vi "RC_Generate_Full_Condition(s)_text.vi"(7 "Array index to show":i32=-1, 8 "error in (no error)":errorcluster, 9 "Array of conditions in":T1, 10 "Calibration parameters":T2 {"True frame time, s" format="%.10g"; "Disp. calibration info"."Speed, µl per ms" format="%.3g"; "True FPS" format="%.10g"; "Timing calibration sw/hw" format="%.10g"}, 11 "TreeControl ref in":refnum<vi>) -> (0 "error out":errorcluster, 3 "TreeControl ref out":refnum<vi>)   [LabVIEW 2018, in "Tracker.lvlib" / "Reward_Condition.lvclass"]
uses:
  Reward_Condition.lvclass
  Controls/CTL_Dispenser_calibration_info.ctl
  Tracker.lvlib
  Controls/CTL_Calibration_parameters.ctl
  Controls/RC_Array_of_Conditions.ctl
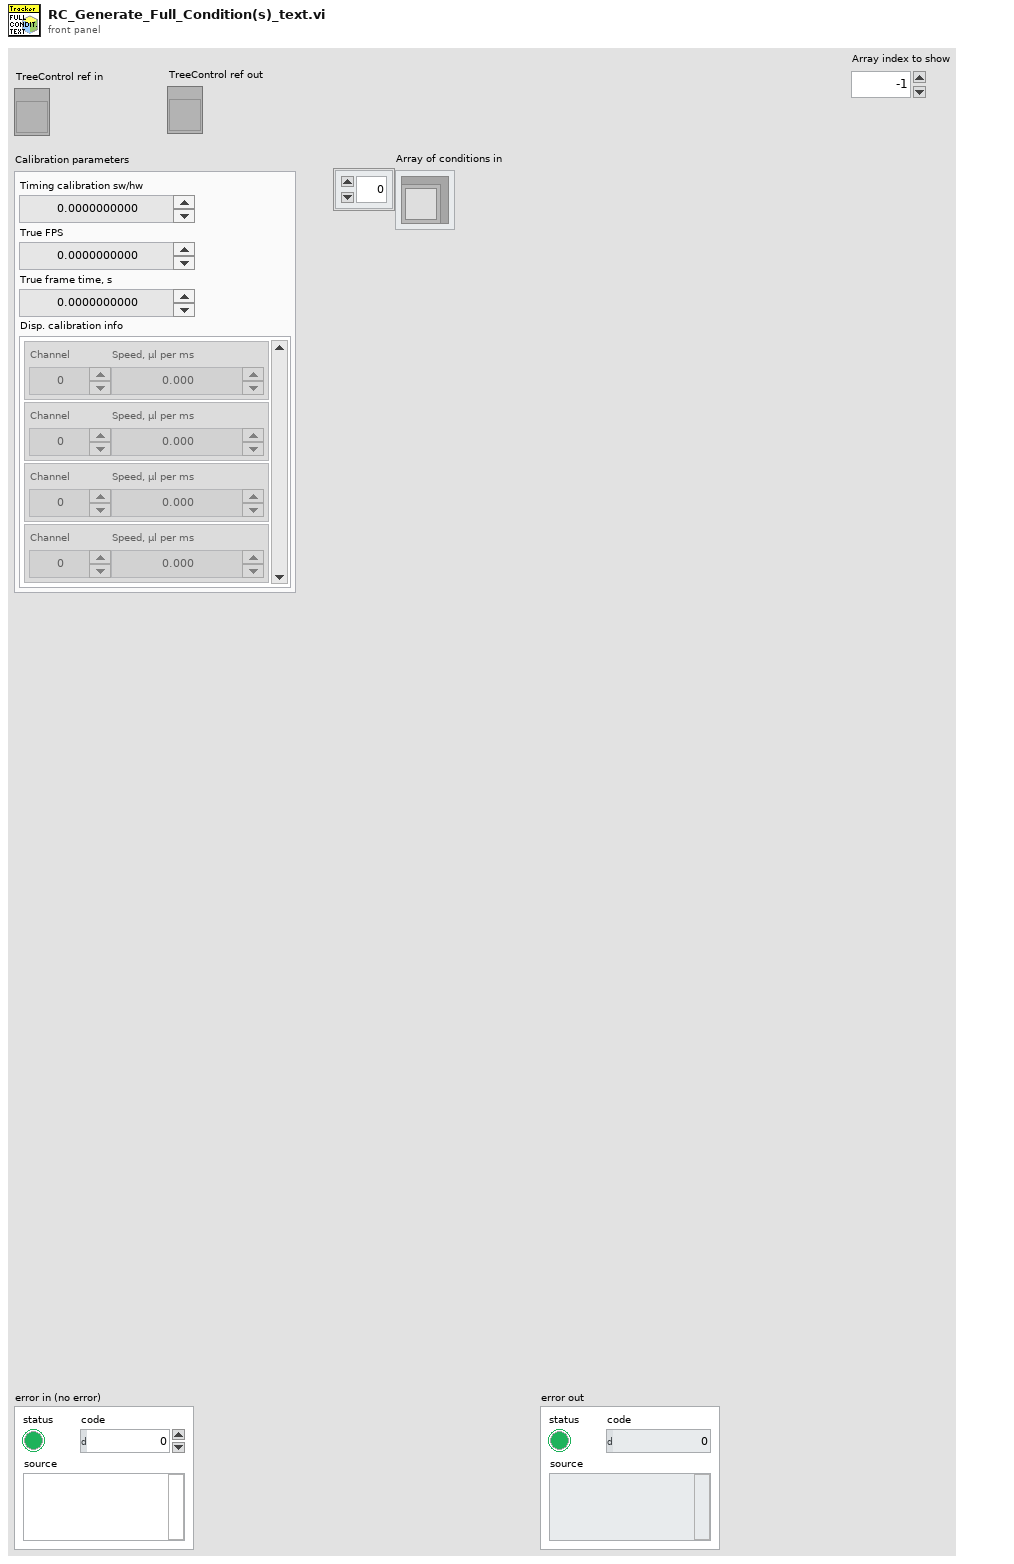
[diagram p1: front panel]
types:
  T1 = typedef "Tracker.lvlib/Reward_Condition.lvclass/RC_Array_of_Conditions.ctl" = refnum<class "Reward_Condition.lvclass">[]
  T2 = typedef "Tracker.lvlib/CTL_Calibration_parameters.ctl" = cluster{"Timing calibration sw/hw":dbl, "True FPS":dbl, "True frame time, s":dbl, "Disp. calibration info":T3}
  T3 = typedef "Tracker.lvlib/CTL_Dispenser_calibration_info.ctl" = cluster{"Channel":u8, "Speed, µl per ms":dbl}[]
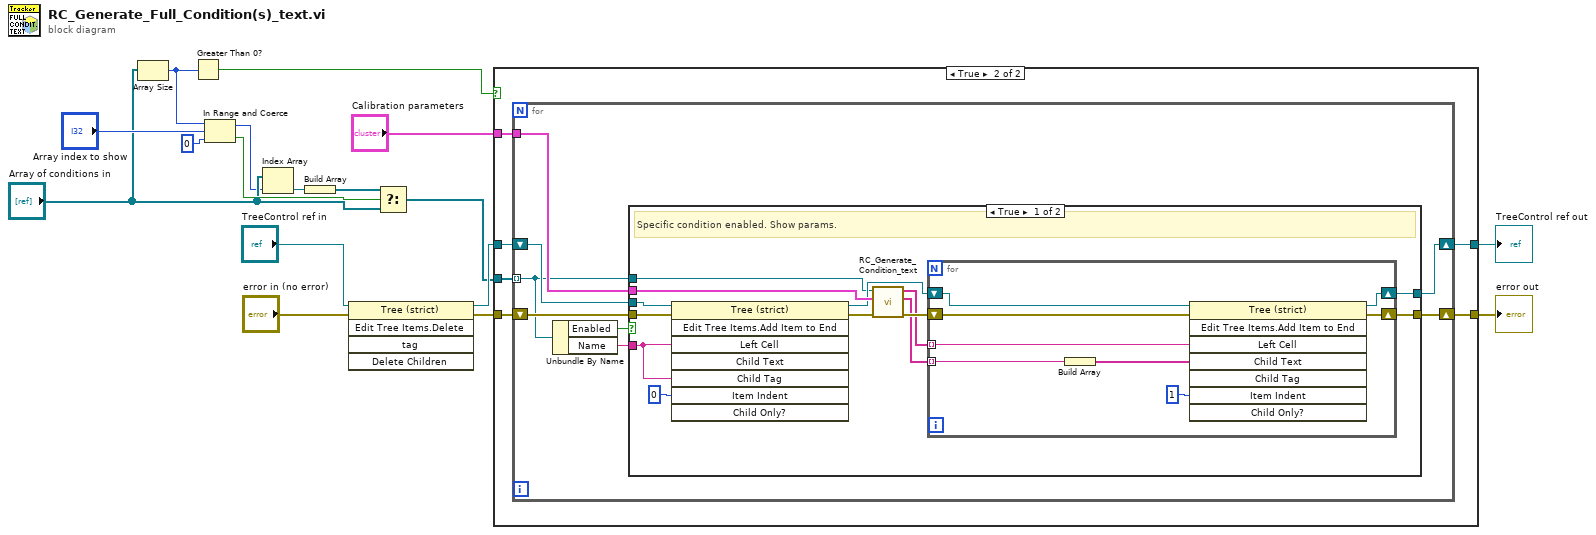
[diagram p0: block diagram]
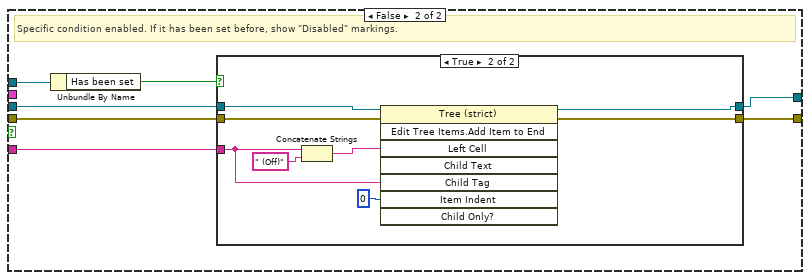
[diagram p3: hidden frame]
diagram:
  n1 = Array Size(array="Array of conditions in") -> (size(s)=w7:i32)
  n2 = Greater Than 0?(x=w7) -> (x > 0?=w13:bool)
  n3 = In Range and Coerce(upper limit=w7, x="Array index to show", lower limit=0) -> (coerced(x)=w3:i32, In Range?=w5:bool)
  n4 = Index Array(array="Array of conditions in", index=w3) -> (element=w2:refnum<class "Reward_Condition.lvclass">)
  n5 = Build Array(w2) -> (w1:refnum<class "Reward_Condition.lvclass">[])
  n6 = invoke on="Invoke Node" class="Tree (strict)" method="Edit Tree Items.Delete"(reference="TreeControl ref in", error in="error in (no error)") -> (reference out=w11:refnum<vi>, error out=w15:errorcluster)  [unwired: 3 in, 3 out]
  n7 = Select(t=w1, s=w5, f="Array of conditions in") -> (s? t:f=w6:T1)
  n8 = case shown="True" w13 {
    tunnel: w6 -> [_ w25]
    tunnel: w15 -> [w19 w24]
    tunnel: [w19 w23] -> w16
    tunnel: "Calibration parameters" -> [_ w22]
    tunnel: w11 -> [w18 w21]
    tunnel: [w18 w20] -> w10
    frame False {
    }
    frame True {
      n9 = for {
        tunnel: w25 -> [w26] mode=indexing
        shift-right: [w31] -> w23
        shift-left: w24 -> [w32]
        tunnel: w22 -> [w29]
        shift-right: [w27] -> w20
        shift-left: w21 -> [w28]
        n10 = Unbundle By Name(w26) -> ("Enabled"=w30:bool, "Name"=w33:string)
        n11 = case shown="True" w30 {
          tunnel: w33 -> [w39 w57]
          tunnel: w32 -> [w46 w61]
          tunnel: [w42 w59] -> w31
          tunnel: w26 -> [w34 w56]
          tunnel: w29 -> [w38 _]
          tunnel: w28 -> [w37 w60]
          tunnel: [w35 w58] -> w27
          frame True {
            # "Specific condition enabled. Show params."
            n12 = invoke on="Invoke Node" class="Tree (strict)" method="Edit Tree Items.Add Item to End"(reference=w37, error in=w46, "Left Cell"=w39, "Child Tag"=w39, "Item Indent"=0 ("New Item Indentation")) -> (reference out=w36:refnum<vi>, error out=w45:errorcluster)  [unwired: 3 in, 6 out]
            n13 = call "RC_Generate_Condition_text.vi"("error in (no error)"=w45, "Calibration parameters"=w38, "Condition in"=w34) -> ("error out"=w43:errorcluster, "Validity criteria"=w40:string[], "SubCondition"=w41:string[])  [unwired: 6 in]
            n14 = for {
              shift-right: [w53] -> w42
              shift-left: w43 -> [w54]
              tunnel: w41 -> [w51] mode=indexing
              tunnel: w40 -> [w50] mode=indexing
              shift-right: [w47] -> w35
              shift-left: w36 -> [w48]
              n15 = Build Array(w50) -> (w49:string[])
              n16 = invoke on="Invoke Node" class="Tree (strict)" method="Edit Tree Items.Add Item to End"(reference=w48, error in=w54, "Left Cell"=w51, "Child Text"=w49, "Item Indent"=1 ("New Item Indentation")) -> (reference out=w47:refnum<vi>, error out=w53:errorcluster)  [unwired: 3 in, 6 out]
            }
          }
          frame False {
            # "Specific condition enabled. If it has been set before, show \"Disabled\" markings."
            n17 = Unbundle By Name(w56) -> ("Has been set"=w55:bool)
            n18 = case shown="True" w55 {
              tunnel: w61 -> [w62 w70]
              tunnel: w60 -> [w63 w69]
              tunnel: [w62 w65] -> w59
              tunnel: [w63 w64] -> w58
              tunnel: w57 -> [_ w68]
              frame False {
              }
              frame True {
                n19 = Concatenate Strings(w68, " (Off)" ("string")) -> (w67:string)
                n20 = invoke on="Invoke Node" class="Tree (strict)" method="Edit Tree Items.Add Item to End"(reference=w69, error in=w70, "Left Cell"=w67, "Child Tag"=w68, "Item Indent"=0 ("New Item Indentation")) -> (reference out=w64:refnum<vi>, error out=w65:errorcluster)  [unwired: 3 in, 6 out]
              }
            }
          }
        }
      }
    }
  }
  "error out" <- w16
  "TreeControl ref out" <- w10
